vi "SerialTest.vi"() -> ()   [LabVIEW 2013]
panel:
  out "#ofPerfectElement":i32
  out "Before":string
  out "After":string
  out "Result":string[](array[string])
  in  "string":string
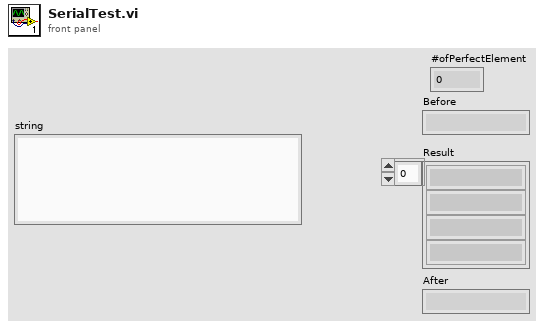
[diagram p1: front panel]
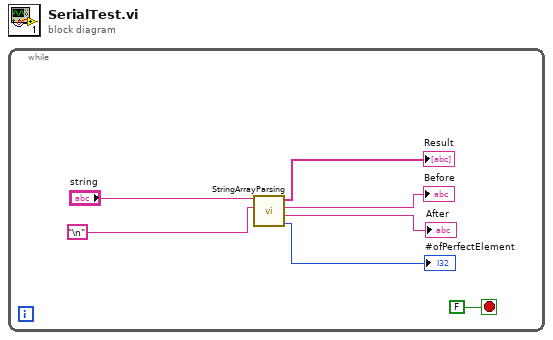
[diagram p0: block diagram]
diagram:
  n1 = while {
    stop <- FALSE stop-if-true
    n2 = call "StringArrayParsing.vi"("delimiter"="\n", "Input String"="string") -> ("#ofPerfectElement"=→"#ofPerfectElement":i32, "After"=→"After":string, "Before"=→"Before":string, "Result"=→"Result":string[])  [unwired: 5 in]
  }
